vi "Init Async Elements.vi"(10 "Async Elements":refnum<queue>) -> (2 "Async Elements":refnum<class "Async Elements.lvclass">)   [LabVIEW 2020, in "jettl.lvlib" / "Base Async Elements.lvlib"]
uses:
  Base Async Elements.lvlib
  Async Elements/Async Elements.lvclass
  Attributes/Attributes.lvclass
  Base Async Elements/Base Async Elements.lvclass
  Async Elements.ctl
  jettl.lvlib
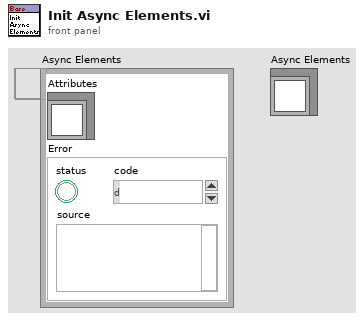
[diagram p1: front panel]
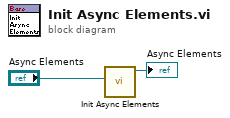
[diagram p0: block diagram]
diagram:
  n1 = call "Init Async Elements.vi"("Async Elements"="Async Elements") -> ("Base Async Elements out"=→"Async Elements":refnum<class "Base Async Elements.lvclass">)  [unwired: 10 in]
